vi "Dropout Voltage.vi"() -> ()   [LabVIEW 2020]
doc: "Demonstrates how to use triggers and events to synchronize multiple channels in Sequence source mode. Use this example to sequence multiple channels in lock-step."
uses:
  <instrlib>/niDCPower/nidcpower.llb/niDCPower Output Function.ctl
  <instrlib>/niDCPower/nidcpower.llb/niDCPower Source Mode.ctl
  <instrlib>/niDCPower/nidcpower.llb/niDCPower Sequence Attribute Type.ctl
  <instrlib>/niDCPower/nidcpower.llb/niDCPower Wait For Event - Event.ctl
  <instrlib>/niDCPower/nidcpower.llb/niDCPower Sense.ctl
  <instrlib>/niDCPower/nidcpower.llb/niDCPower Create Advanced Sequence Step.vi
  <instrlib>/niDCPower/nidcpower.llb/niDCPower Disable Source Trigger.vi
  <instrlib>/niDCPower/nidcpower.llb/niDCPower Configure Digital Edge Source Trigger.vi
  <instrlib>/niDCPower/nidcpower.llb/niDCPower Configure Digital Edge Measure Trigger.vi
panel:
  in  "Aperture time (s)":dbl=0.1
  in  "DUT setup time (s)":dbl
  out "Input Voltage (V) vs. Output Voltage (V)":T1(graph) caption="Current (Amps) vs Voltage (Volts)"
  in  "Load device wait (s)":dbl=0.1
  in  "Sweep type":u16(ring) items=["Linear", "Logarithmic"]
  in  "Load device max. voltage (V)":dbl=20.0
  in  "Load values (A)":dbl[](array[numeric])=[0.01, 0.1, 1.0, 2.5] min=0.0
  in  "Timeout (s)":dbl=30.0 format="%.3p"
  in  "Source device name":refnum<k15>="PXI2Slot2"
  in  "Load device source delay (s)":dbl=0.1
  in  "Source device current limit (A)":dbl=25.0
  in  "Load device max. sink power (W)":dbl=300.0
  in  "Source device channel":string="0"
  in  "Load device channel":string="0"
  in  "Points or Points/Decade":i32=21 min=1
  in  "Voltage source level stop":dbl=3.0 caption="Current load level stop" min=0.0 step=0.1
  in  "Voltage source level start":dbl=6.5 min=0.0 step=0.1
  in  "Load device name":refnum<k15>="PXI2Slot4"
  # "Source config"
  # "Load Config"
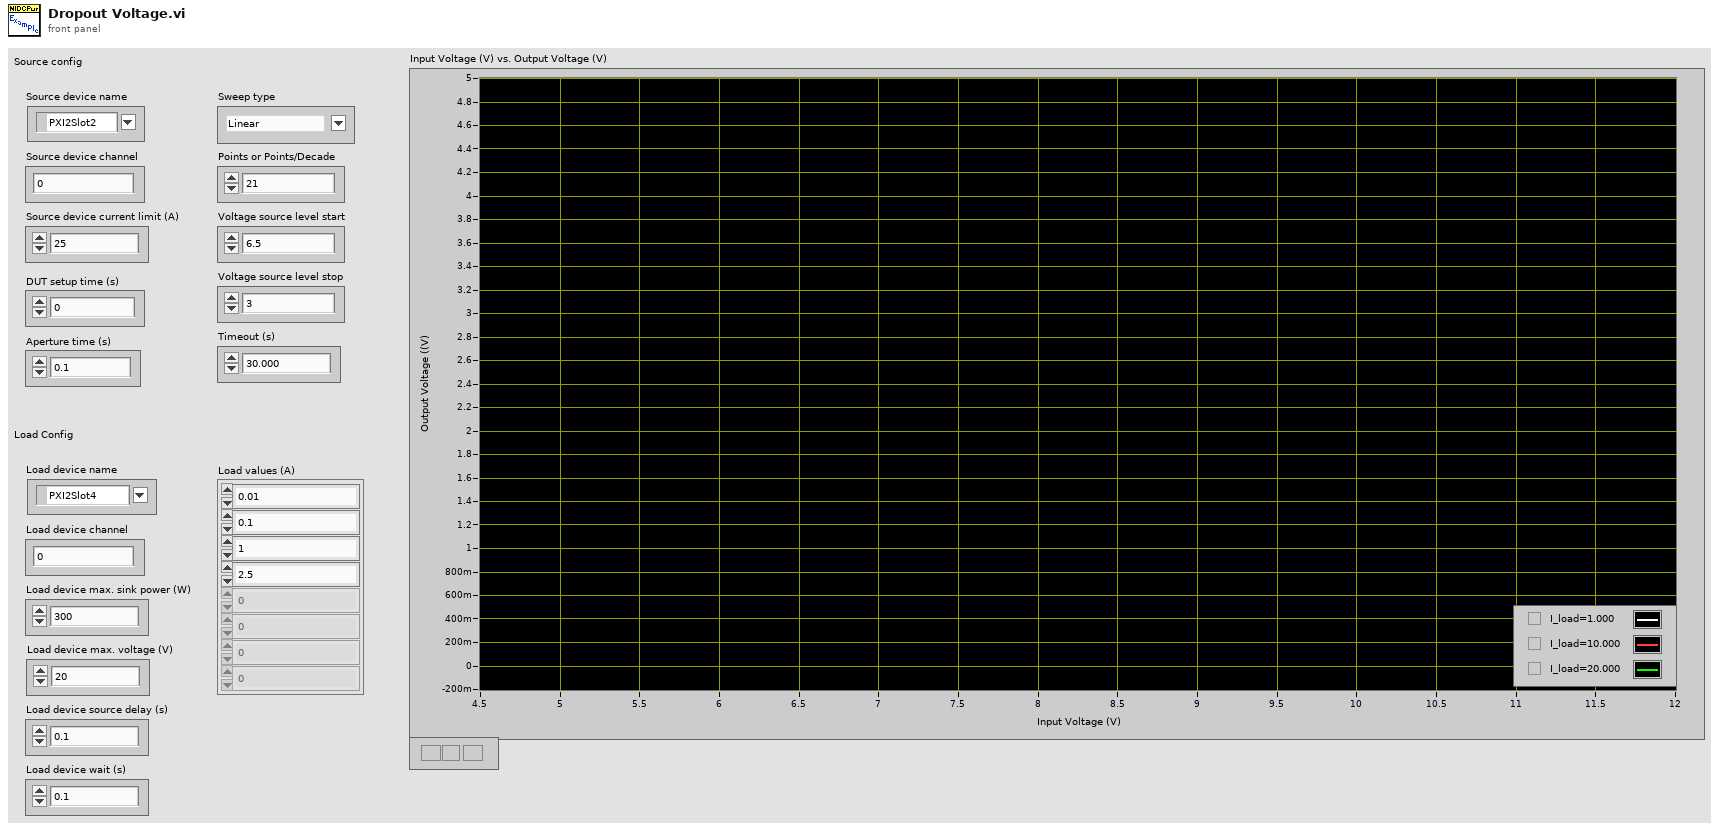
[diagram p1: front panel]
types:
  T1 = cluster{"voltage measurements":dbl[], "current measurements":dbl[]}[]
  T2 = typedef "niDCPower Wait For Event - Event.ctl" = i32
  T3 = typedef "niDCPower Source Mode.ctl" = i32
  T4 = typedef "niDCPower Sense.ctl" = i32
  T5 = typedef "niDCPower Sequence Attribute Type.ctl" = i32
  T6 = typedef "niDCPower Output Function.ctl" = i32
  T7 = cluster{"voltage measurements":dbl[], "voltage measurements":dbl[]}
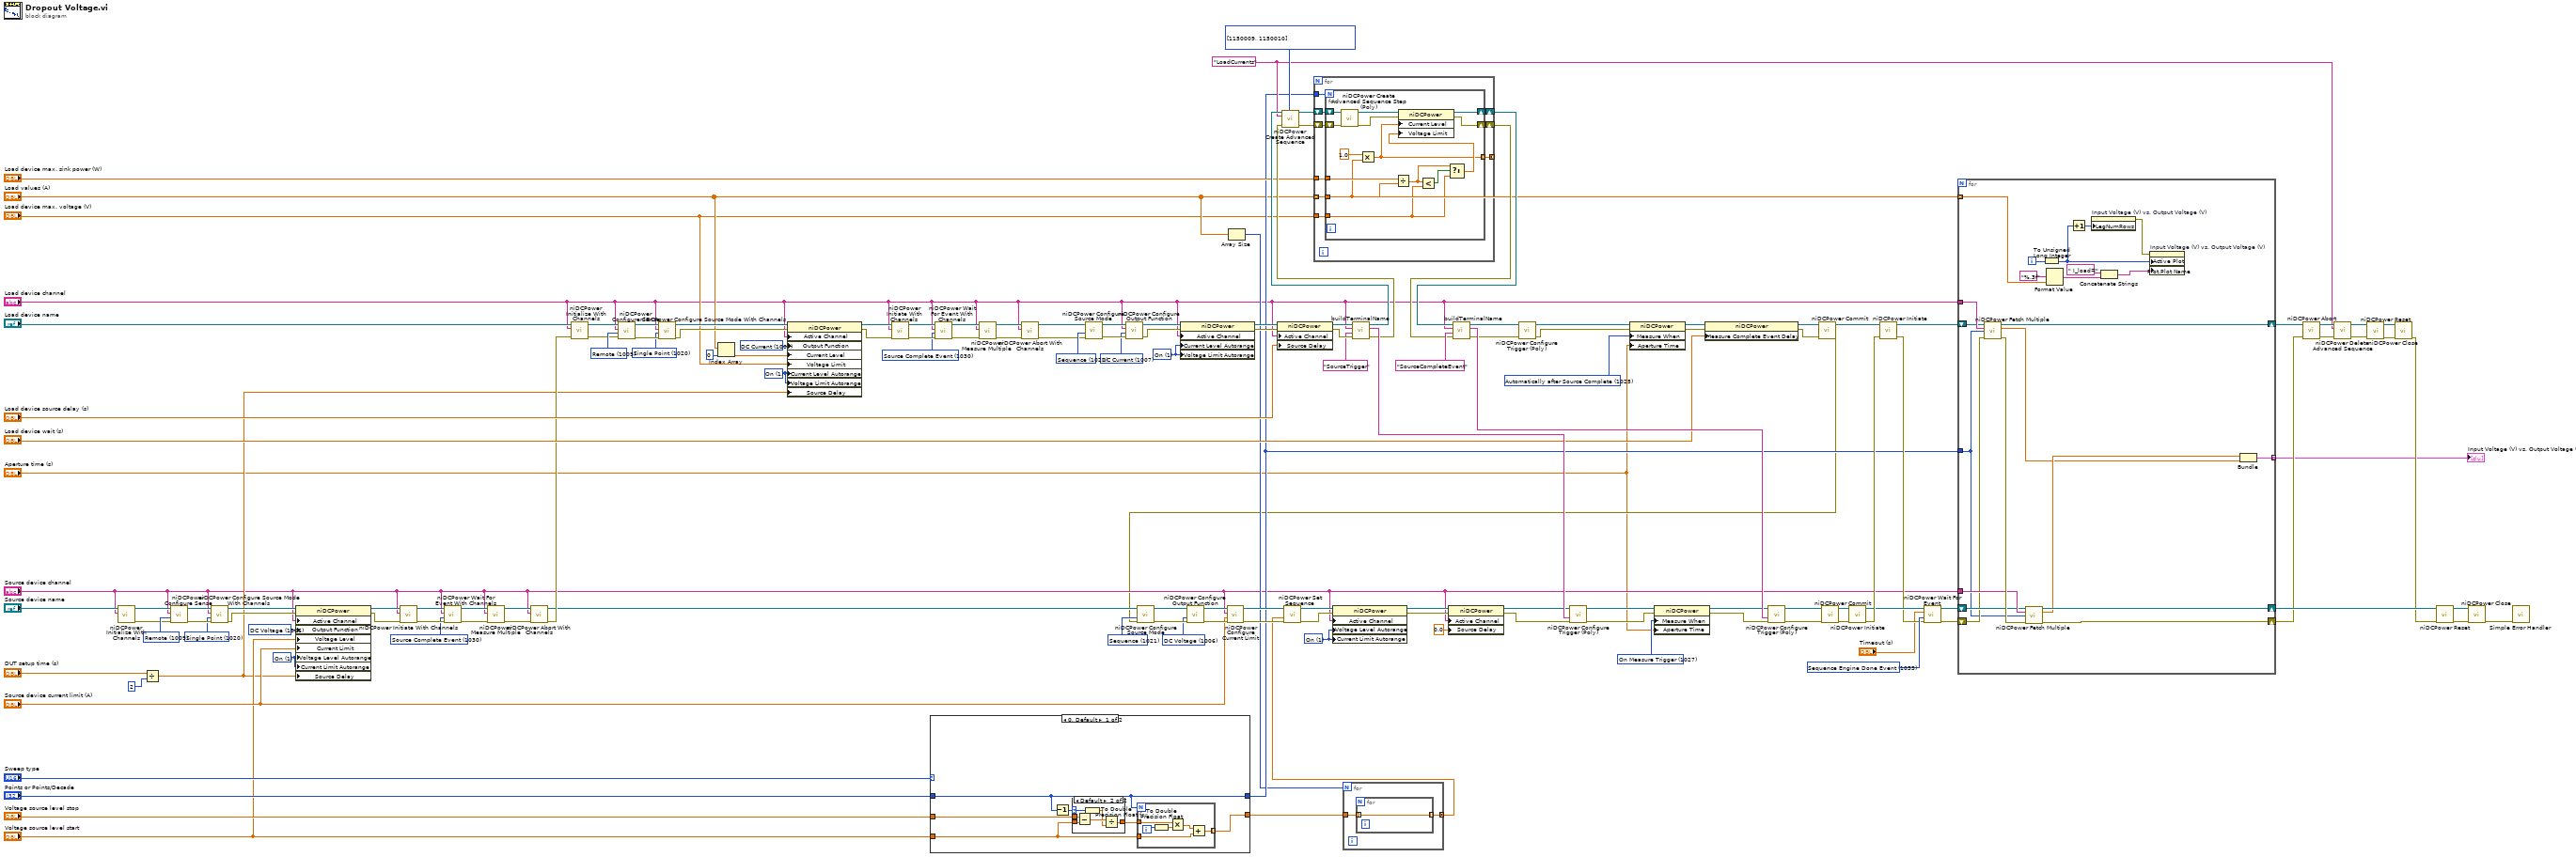
[diagram p0: block diagram]
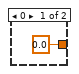
[diagram p2: hidden frame]
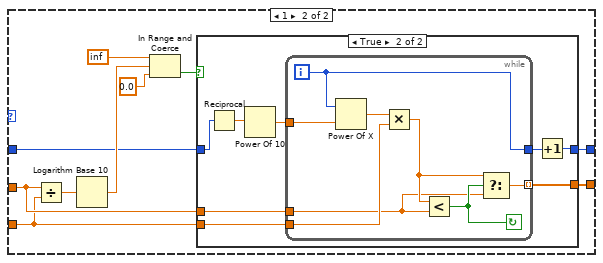
[diagram p3: hidden frame]
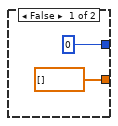
[diagram p4: hidden frame]
diagram:
  w1 = 1025 items=["Automatically after Source Complete"=1025, "On Demand"=1026, "On Measure Trigger"=1027] ("Measurement:Advanced:Measure When")
  w20 = T2 1030 items=["Source Complete Event"=1030, "Measure Complete Event"=1031, "Sequence Iteration Complete Event"=1032, "Sequence Engine Done Event"=1033, "Pulse Complete Event"=1051, "Ready For Pulse Trigger Event"=1052] ("event")
  w25 = 1 items=["Off", "On"] ("Source:DC Current:Current Level Autorange")
  w26 = 1007 items=["DC Voltage"=1006, "DC Current"=1007, "Pulse Voltage"=1049, "Pulse Current"=1050] ("Source:Output Function")
  w27 = T3 1020 items=["Single Point"=1020, "Sequence"=1021] ("source mode")
  w32 = T4 1009 items=["Local"=1008, "Remote"=1009] ("sense")
  w44 = T2 1030 items=["Source Complete Event"=1030, "Measure Complete Event"=1031, "Sequence Iteration Complete Event"=1032, "Sequence Engine Done Event"=1033, "Pulse Complete Event"=1051, "Ready For Pulse Trigger Event"=1052] ("event")
  w49 = 1 items=["Off", "On"] ("Source:DC Current:Current Level Autorange")
  w50 = 1006 items=["DC Voltage"=1006, "DC Current"=1007, "Pulse Voltage"=1049, "Pulse Current"=1050] ("Source:Output Function")
  w51 = T3 1020 items=["Single Point"=1020, "Sequence"=1021] ("source mode")
  w56 = T4 1009 items=["Local"=1008, "Remote"=1009] ("sense")
  w91 = T2 1033 items=["Source Complete Event"=1030, "Measure Complete Event"=1031, "Sequence Iteration Complete Event"=1032, "Sequence Engine Done Event"=1033] ("event")
  w96 = 1 items=["Off", "On"] ("DC Voltage:Voltage Level Autorange")
  w110 = 1 items=["Off", "On"] ("DC Voltage:Voltage Level Autorange")
  w111 = T5[] [1150009, 1150010] items=["Source -> Output Function"=1150008, "Source -> Output Enabled"=1250006, "Source -> Output Resistance"=1150061, "Source -> Transient Response"=1150062, "Source -> Custom Transient Response -> Voltage Gain Bandwidth"=1150067, "Source -> Custom Transient Response -> Voltage Compensation Frequency"=1150068, "Source -> Custom Transient Response -> Voltage Pole-Zero Ratio"=1150069, "Source -> Custom Transient Response -> Current Gain Bandwidth"=1150070, "Source -> Custom Transient Response -> Current Compensation Frequency"=1150071, "Source -> Custom Transient Response -> Current Pole-Zero Ratio"=1150072, "Source -> DC Voltage -> Voltage Level"=1250001, "Source -> DC Voltage -> Voltage Level Range"=1150005, "Source -> DC Voltage -> Current Limit"=1250005, "Source -> DC Voltage -> Current Limit High"=1150187, "Source -> DC Voltage -> Current Limit Low"=1150188, "Source -> DC Voltage -> Current Limit Range"=1150004, "Source -> DC Current -> Current Level"=1150009, "Source -> DC Current -> Current Level Range"=1150011, "Source -> DC Current -> Voltage Limit"=1150010, "Source -> DC Current -> Voltage Limit High"=1150185, "Source -> DC Current -> Voltage Limit Low"=1150186, "Source -> DC Current -> Voltage Limit Range"=1150012, "Source -> Pulse Voltage -> Pulse Voltage Level"=1150080, "Source -> Pulse Voltage -> Pulse Bias Voltage Level"=1150082, "Source -> Pulse Voltage -> Pulse Voltage Level Range"=1150084, "Source -> Pulse Voltage -> Pulse Current Limit"=1150081, "Source -> Pulse Voltage -> Pulse Current Limit High"=1150193, "Source -> Pulse Voltage -> Pulse Current Limit Low"=1150194, "Source -> Pulse Voltage -> Pulse Bias Current Limit"=1150083, "Source -> Pulse Voltage -> Pulse Bias Current Limit High"=1150195, "Source -> Pulse Voltage -> Pulse Bias Current Limit Low"=1150196, "Source -> Pulse Voltage -> Pulse Current Limit Range"=1150085, "Source -> Pulse Current -> Pulse Current Level"=1150086, "Source -> Pulse Current -> Pulse Bias Current Level"=1150088, "Source -> Pulse Current -> Pulse Current Level Range"=1150090, "Source -> Pulse Current -> Pulse Voltage Limit"=1150087, "Source -> Pulse Current -> Pulse Voltage Limit High"=1150189, "Source -> Pulse Current -> Pulse Voltage Limit Low"=1150190, "Source -> Pulse Current -> Pulse Bias Voltage Limit"=1150089, "Source -> Pulse Current -> Pulse Bias Voltage Limit High"=1150191, "Source -> Pulse Current -> Pulse Bias Voltage Limit Low"=1150192, "Source -> Pulse Current -> Pulse Voltage Limit Range"=1150091, "Source -> Advanced -> Source Delay"=1150051, "Source -> Advanced -> Pulse Bias Delay"=1150092, "Source -> Advanced -> Pulse On Time"=1150093, "Source -> Advanced -> Pulse Off Time"=1150094, "Source -> Advanced -> OVP Enabled"=1250002, "Source -> Advanced -> OVP Limit"=1250003, "Source -> Advanced -> Compliance Limit Symmetry"=1150184, "Source -> Advanced -> Sequence Step Delta Time"=1150198, "Measurement -> Sense"=1150013, "Measurement -> Aperture Time"=1150058, "Measurement -> Measure Record Length"=1150063, "Measurement -> Advanced -> DC Noise Rejection"=1150066, "Measurement -> Autorange"=1150244, "Measurement -> Advanced -> Autorange Behavior"=1150245, "Measurement -> Advanced -> Autorange Aperture Time Mode"=1150246, "Measurement -> Advanced -> Autorange Minimum Aperture Time"=1150247, "Measurement -> Advanced -> Autorange Minimum Aperture Time Units"=1150248, "Measurement -> Advanced -> Autorange Minimum Current Range"=1150255, "Measurement -> Advanced -> Autorange Minimum Voltage Range"=1150256, "Measurement -> Advanced -> Autorange Threshold Mode"=1150257, "Measurement -> Advanced -> Autorange Maximum Delay After Range Change"=1150322, "LCR -> Instrument Mode"=1150208, "LCR -> LCR Stimulus Function"=1150209, "LCR -> LCR Frequency"=1150210, "LCR -> LCR Voltage Amplitude"=1150211, "LCR -> LCR Current Amplitude"=1150212, "LCR -> LCR DC Bias Source"=1150213, "LCR -> LCR DC Bias Voltage Level"=1150214, "LCR -> LCR DC Bias Current Level"=1150215, "LCR -> LCR Impedance Autorange"=1150216, "LCR -> LCR Impedance Range"=1150217, "LCR -> LCR Measurement Time"=1150218, "LCR -> LCR Custom Measurement Time"=1150258, "LCR -> LCR Source Delay Mode"=1150315, "LCR -> Compensation -> Open -> Enabled"=1150220, "LCR -> Compensation -> Open -> Conductance"=1150261, "LCR -> Compensation -> Open -> Susceptance"=1150262, "LCR -> Compensation -> Short -> Enabled"=1150221, "LCR -> Compensation -> Short -> Resistance"=1150263, "LCR -> Compensation -> Short -> Reactance"=1150264, "LCR -> Compensation -> Load -> Enabled"=1150222, "LCR -> Compensation -> Load -> Measured Resistance"=1150268, "LCR -> Compensation -> Load -> Measured Reactance"=1150269, "LCR -> Compensation -> Load -> Actual Resistance"=1150270, "LCR -> Compensation -> Load -> Actual Reactance"=1150271] ("advanced sequence properties")
  w76 = "LoadCurrents" ("sequence name")
  w116 = T6 1006 items=["DC Voltage"=1006, "DC Current"=1007, "Pulse Voltage"=1049, "Pulse Current"=1050] ("output function")
  w117 = 1027 items=["Automatically after Source Complete"=1025, "On Demand"=1026, "On Measure Trigger"=1027] ("Measurement:Advanced:Measure When")
  w118 = T3 1021 items=["Single Point"=1020, "Sequence"=1021] ("source mode")
  w125 = T6 1007 items=["DC Voltage"=1006, "DC Current"=1007, "Pulse Voltage"=1049, "Pulse Current"=1050] ("output function")
  w139 = T3 1021 items=["Single Point"=1020, "Sequence"=1021] ("source mode")
  n1 = call <instrlib>:"niDCPower Initialize With Channels.vi"("channels"="Source device channel", "resource name"="Source device name") -> ("error out"=w37:errorcluster, "instrument handle out"=w38:refnum<k15>)  [unwired: 3 in, 5 out]
  n2 = Divide(x="DUT setup time (s)", y=2) -> (x/y=w12:dbl)
  n3 = call <instrlib>:"niDCPower Configure Sense.vi"("error in (no error)"=w37, "sense"=w56, "channel name"="Source device channel", "instrument handle"=w38) -> ("error out"=w52:errorcluster, "instrument handle out"=w53:refnum<k15>)  [unwired: 6 in]
  n4 = call <instrlib>:"niDCPower Configure Source Mode With Channels.vi"("error in (no error)"=w52, "source mode"=w51, "channel name"="Source device channel", "instrument handle"=w53) -> ("error out"=w55:errorcluster, "instrument handle out"=w54:refnum<k15>)  [unwired: 6 in]
  n5 = property class="niDCPower"(reference=w54, error in=w55, "Active Channel"="Source device channel", "Output Function"=w50, "Voltage Level"="Voltage source level start", "Current Limit"="Source device current limit (A)", "Voltage Level Autorange"=w49, "Current Limit Autorange"=w49, "Source Delay"=w12) -> (reference out=w48:refnum<k15>, error out=w47:errorcluster)
  n6 = call <instrlib>:"niDCPower Initiate With Channels.vi"("error in (no error)"=w47, "channel name"="Source device channel", "instrument handle"=w48) -> ("error out"=w45:errorcluster, "instrument handle out"=w46:refnum<k15>)  [unwired: 7 in]
  n7 = call <instrlib>:"niDCPower Wait For Event With Channels.vi"("error in (no error)"=w45, "event"=w44, "channel name"="Source device channel", "instrument handle"=w46) -> ("error out"=w43:errorcluster, "instrument handle out"=w42:refnum<k15>)  [unwired: 6 in]
  n8 = call <instrlib>:"niDCPower Measure Multiple.vi"("error in (no error)"=w43, "channel name"="Source device channel", "instrument handle"=w42) -> ("error out"=w40:errorcluster, "instrument handle out"=w39:refnum<k15>)  [unwired: 5 in, 2 out]
  n9 = call <instrlib>:"niDCPower Abort With Channels.vi"("error in (no error)"=w40, "channel name"="Source device channel", "instrument handle"=w39) -> ("error out"=w33:errorcluster, "instrument handle out"=w6:refnum<k15>)  [unwired: 7 in]
  n10 = call <instrlib>:"niDCPower Initialize With Channels.vi"("error in (no error)"=w33, "channels"="Load device channel", "resource name"="Load device name") -> ("error out"=w13:errorcluster, "instrument handle out"=w14:refnum<k15>)  [unwired: 2 in, 5 out]
  n11 = call <instrlib>:"niDCPower Configure Sense.vi"("error in (no error)"=w13, "sense"=w32, "channel name"="Load device channel", "instrument handle"=w14) -> ("error out"=w28:errorcluster, "instrument handle out"=w29:refnum<k15>)  [unwired: 6 in]
  n12 = call <instrlib>:"niDCPower Configure Source Mode With Channels.vi"("error in (no error)"=w28, "source mode"=w27, "channel name"="Load device channel", "instrument handle"=w29) -> ("error out"=w31:errorcluster, "instrument handle out"=w30:refnum<k15>)  [unwired: 6 in]
  n13 = Index Array(array="Load values (A)", index=0) -> (element=w10:dbl)
  n14 = property class="niDCPower"(reference=w30, error in=w31, "Active Channel"="Load device channel", "Output Function"=w26, "Current Level"=w10, "Voltage Limit"="Load device max. voltage (V)", "Current Level Autorange"=w25, "Voltage Limit Autorange"=w25, "Source Delay"=w12) -> (reference out=w24:refnum<k15>, error out=w23:errorcluster)
  n15 = call <instrlib>:"niDCPower Initiate With Channels.vi"("error in (no error)"=w23, "channel name"="Load device channel", "instrument handle"=w24) -> ("error out"=w21:errorcluster, "instrument handle out"=w22:refnum<k15>)  [unwired: 7 in]
  n16 = case shown="0, Default" "Sweep type" {
    tunnel: "Points or Points/Decade" -> [w148 w167]
    tunnel: [w151 w171] -> w61
    tunnel: "Voltage source level start" -> [w150 w168]
    tunnel: "Voltage source level stop" -> [w149 w175]
    tunnel: [w148 w172] -> w73
    frame 0, Default {
      n17 = Decrement(x=w148) -> (x-1=w153:i32)
      n18 = case shown="Default" w153 {
        selector: w153 -> [_ w161]
        tunnel: w149 -> [_ w166]
        tunnel: w150 -> [_ w165]
        tunnel: [0.0 w163] -> w152
        frame 0 {
        }
        frame Default {
          n19 = Subtract(x=w166, y=w165) -> (x-y=w164:dbl)
          n20 = To Double Precision Float(number=w161) -> (double precision float=w162:dbl)
          n21 = Divide(x=w164, y=w162) -> (x/y=w163:dbl)
        }
      }
      n22 = for {
        N: w148 -> [_]
        tunnel: w152 -> [w158]
        tunnel: w150 -> [w159]
        tunnel: [w154] -> w151 mode=indexing
        i -> [w157]
        n23 = To Double Precision Float(number=w157) -> (double precision float=w155:dbl)
        n24 = Multiply(x=w158, y=w155) -> (x*y=w156:dbl)
        n25 = Add(x=w156, y=w159) -> (x+y=w154:dbl)
      }
    }
    frame 1 {
      n26 = Divide(x=w175, y=w168) -> (x/y=w176:dbl)
      n27 = Logarithm Base 10(1:w176) -> (0:w173:dbl)
      n28 = In Range and Coerce(upper limit=inf, x=w173, lower limit=0.0) -> (In Range?=w170:bool)  [unwired: 1 out]
      n29 = case shown="True" w170 {
        tunnel: [dbl[] [] w186] -> w171
        tunnel: [0 w179] -> w172
        tunnel: w175 -> [_ w185]
        tunnel: w168 -> [_ w184]
        tunnel: w167 -> [_ w181]
        frame False {
        }
        frame True {
          n30 = Reciprocal(x=w181) -> (1/x=w183:dbl)
          n31 = Power Of 10(x=w183) -> (10^x=w182:dbl)
          n32 = while {
            tunnel: w182 -> [w191]
            tunnel: w184 -> [w194]
            tunnel: [w190] -> w186 mode=indexing
            tunnel: [w192] -> w180
            tunnel: w185 -> [w187]
            i -> [w192]
            stop <- w189 continue-if-true
            n33 = Power Of X(1:w191, 2:w192) -> (0:w193:dbl)
            n34 = Multiply(x=w193, y=w194) -> (x*y=w188:dbl)
            n35 = Less?(x=w188, y=w187) -> (x < y?=w189:bool)
            n36 = Select(t=w188, s=w189, f=w187) -> (s? t:f=w190:dbl)
          }
          n37 = Increment(x=w180) -> (x+1=w179:i32)
        }
      }
    }
  }
  n38 = call <instrlib>:"niDCPower Wait For Event With Channels.vi"("error in (no error)"=w21, "event"=w20, "channel name"="Load device channel", "instrument handle"=w22) -> ("error out"=w19:errorcluster, "instrument handle out"=w18:refnum<k15>)  [unwired: 6 in]
  n39 = call <instrlib>:"niDCPower Measure Multiple.vi"("error in (no error)"=w19, "channel name"="Load device channel", "instrument handle"=w18) -> ("error out"=w17:errorcluster, "instrument handle out"=w16:refnum<k15>)  [unwired: 5 in, 2 out]
  n40 = call <instrlib>:"niDCPower Abort With Channels.vi"("error in (no error)"=w17, "channel name"="Load device channel", "instrument handle"=w16) -> ("error out"=w7:errorcluster, "instrument handle out"=w8:refnum<k15>)  [unwired: 7 in]
  n41 = call <instrlib>:"niDCPower Configure Source Mode.vi"("error in (no error)"=w7, "source mode"=w139, "instrument handle"=w8) -> ("error out"=w141:errorcluster, "instrument handle out"=w140:refnum<k15>)  [unwired: 7 out]
  n42 = call <instrlib>:"niDCPower Configure Output Function.vi"("error in (no error)"=w141, "output function"=w125, "channel name"="Load device channel", "instrument handle"=w140) -> ("error out"=w57:errorcluster, "instrument handle out"=w58:refnum<k15>)  [unwired: 6 out]
  n43 = property class="niDCPower"(reference=w58, error in=w57, "Active Channel"="Load device channel", "Current Level Autorange"=w110, "Voltage Limit Autorange"=w110) -> (reference out=w108:refnum<k15>, error out=w107:errorcluster)
  n44 = Array Size(array="Load values (A)") -> (size(s)=w66:i32)
  n45 = property class="niDCPower"(reference=w108, error in=w107, "Active Channel"="Load device channel", "Source Delay"="Load device source delay (s)") -> (reference out=w133:refnum<k15>, error out=w131:errorcluster)
  n46 = for {
    N: w66 -> [_]
    tunnel: w61 -> [w196]
    tunnel: [w195] -> w67 mode=concatenating
    n47 = for {
      tunnel: w196 -> [w197] mode=indexing
      tunnel: [w197] -> w195 mode=indexing
    }
  }
  n48 = call "buildTerminalName.vi"("error in (no error)"=w131, "Local Terminal Name"="SourceTrigger", "Channel Name"="Load device channel", "session handle"=w133) -> ("error IO"=w103:errorcluster, "Fully Qualified Terminal Name"=w129:string, "session handle 2"=w105:refnum<k15>)  [unwired: 5 out]
  n49 = call <instrlib>:"niDCPower Create Advanced Sequence.vi"("instrument handle"=w105, "sequence name"=w76, "advanced sequence properties"=w111, "error in (no error)"=w103) -> ("instrument handle out"=w113:refnum<k15>, "error out"=w112:errorcluster)  [unwired: 10 in]
  n50 = for {
    tunnel: "Load device max. sink power (W)" -> [w202]
    tunnel: "Load device max. voltage (V)" -> [w201]
    tunnel: "Load values (A)" -> [w200] mode=indexing
    shift-right: [w204] -> w104
    shift-left: w113 -> [w206]
    shift-right: [w203] -> w102
    shift-left: w112 -> [w205]
    tunnel: w73 -> [w199]
    tunnel: [w198] -> _ mode=concatenating
    n51 = for {
      N: w199 -> [_]
      shift-right: [w217] -> w203
      shift-left: w205 -> [w220]
      shift-right: [w216] -> w204
      shift-left: w206 -> [w215]
      tunnel: w202 -> [w214]
      tunnel: w200 -> [w209]
      tunnel: w201 -> [w212]
      tunnel: [w207] -> w198 mode=indexing
      n52 = call-poly <instrlib>:"niDCPower Create Advanced Sequence Step (Poly).vi"("error in (no error)"=w220, "instrument handle"=w215) -> ("error out"=w218:errorcluster, "instrument handle out"=w219:refnum<k15>)  [unwired: 8 in]
      n53 = Multiply(x=1.0, y=w209) -> (x*y=w207:dbl)
      n54 = Divide(x=w214, y=w209) -> (x/y=w211:dbl)
      n55 = Less?(x=w211, y=w212) -> (x < y?=w213:bool)
      n56 = Select(t=w211, s=w213, f=w212) -> (s? t:f=w210:dbl)
      n57 = property class="niDCPower"(reference=w219, error in=w218, "Current Level"=w207, "Voltage Limit"=w210) -> (reference out=w216:refnum<k15>, error out=w217:errorcluster)
    }
  }
  n58 = call "buildTerminalName.vi"("error in (no error)"=w102, "Local Terminal Name"="SourceCompleteEvent", "Channel Name"="Load device channel", "session handle"=w104) -> ("error IO"=w127:errorcluster, "Fully Qualified Terminal Name"=w128:string, "session handle 2"=w132:refnum<k15>)  [unwired: 5 out]
  n59 = call-poly <instrlib>:"niDCPower Configure Trigger (Poly).vi"("error in (no error)"=w127, "instrument handle"=w132) -> ("error out"=w142:errorcluster, "instrument handle out"=w143:refnum<k15>)  [unwired: 1 in, 7 out]
  n60 = property class="niDCPower"(reference=w143, error in=w142, "Measure When"=w1, "Aperture Time"="Aperture time (s)") -> (reference out=w137:refnum<k15>, error out=w134:errorcluster)
  n61 = property class="niDCPower"(reference=w137, error in=w134, "Measure Complete Event Delay"="Load device wait (s)") -> (reference out=w136:refnum<k15>, error out=w135:errorcluster)
  n62 = call <instrlib>:"niDCPower Commit.vi"("error in (no error)"=w135, "instrument handle"=w136) -> ("error out"=w3:errorcluster, "instrument handle out"=w63:refnum<k15>)  [unwired: 8 out]
  n63 = call <instrlib>:"niDCPower Configure Source Mode.vi"("error in (no error)"=w3, "source mode"=w118, "instrument handle"=w6) -> ("error out"=w120:errorcluster, "instrument handle out"=w119:refnum<k15>)  [unwired: 7 out]
  n64 = call <instrlib>:"niDCPower Configure Output Function.vi"("error in (no error)"=w120, "output function"=w116, "instrument handle"=w119) -> ("error out"=w60:errorcluster, "instrument handle out"=w59:refnum<k15>)  [unwired: 1 in, 6 out]
  n65 = call <instrlib>:"niDCPower Configure Current Limit.vi"("error in (no error)"=w60, "current limit"="Source device current limit (A)", "channel name"="Source device channel", "instrument handle"=w59) -> ("error out"=w92:errorcluster, "instrument handle out"=w93:refnum<k15>)  [unwired: 6 in]
  n66 = call <instrlib>:"niDCPower Set Sequence.vi"("error in (no error)"=w92, "values"=w67, "instrument handle"=w93) -> ("error out"=w68:errorcluster, "instrument handle out"=w69:refnum<k15>)  [unwired: 2 in, 5 out]
  n67 = property class="niDCPower"(reference=w69, error in=w68, "Active Channel"="Source device channel", "Voltage Level Autorange"=w96, "Current Limit Autorange"=w96) -> (reference out=w95:refnum<k15>, error out=w94:errorcluster)
  n68 = property class="niDCPower"(reference=w95, error in=w94, "Active Channel"="Source device channel", "Source Delay"=0.0 ("Source:Advanced:Source Delay")) -> (reference out=w71:refnum<k15>, error out=w70:errorcluster)
  n69 = call-poly <instrlib>:"niDCPower Configure Trigger (Poly).vi"("error in (no error)"=w70, "input terminal"=w129, "instrument handle"=w71) -> ("error out"=w123:errorcluster, "instrument handle out"=w124:refnum<k15>)  [unwired: 1 in, 6 out]
  n70 = property class="niDCPower"(reference=w124, error in=w123, "Measure When"=w117, "Aperture Time"="Aperture time (s)") -> (reference out=w121:refnum<k15>, error out=w122:errorcluster)
  n71 = call-poly <instrlib>:"niDCPower Configure Trigger (Poly).vi"("error in (no error)"=w122, "input terminal"=w128, "instrument handle"=w121) -> ("error out"=w65:errorcluster, "instrument handle out"=w64:refnum<k15>)  [unwired: 1 in, 6 out]
  n72 = call <instrlib>:"niDCPower Commit.vi"("error in (no error)"=w65, "instrument handle"=w64) -> ("error out"=w145:errorcluster, "instrument handle out"=w146:refnum<k15>)  [unwired: 8 out]
  n73 = call <instrlib>:"niDCPower Initiate.vi"("error in (no error)"=w145, "instrument handle"=w146) -> ("error out"=w138:errorcluster, "instrument handle out"=w90:refnum<k15>)  [unwired: 8 out]
  n74 = call <instrlib>:"niDCPower Initiate.vi"("error in (no error)"=w138, "instrument handle"=w63) -> ("error out"=w88:errorcluster, "instrument handle out"=w86:refnum<k15>)  [unwired: 8 out]
  n75 = call <instrlib>:"niDCPower Wait For Event.vi"("timeout (10.0)"="Timeout (s)", "error in (no error)"=w88, "event"=w91, "instrument handle"=w90) -> ("error out"=w87:errorcluster, "instrument handle out"=w89:refnum<k15>)  [unwired: 6 out]
  n76 = for {
    tunnel: "Source device channel" -> [w240]
    tunnel: "Load device channel" -> [w239]
    shift-right: [w242] -> w144
    shift-left: w89 -> [w238]
    shift-right: [w234] -> w78
    shift-left: w87 -> [w237]
    shift-right: [w235] -> w79
    shift-left: w86 -> [w236]
    tunnel: w73 -> [w223]
    tunnel: "Load values (A)" -> [w230] mode=indexing
    tunnel: [w224] -> w75 mode=indexing
    i -> [w225]
    n77 = call <instrlib>:"niDCPower Fetch Multiple.vi"("instrument handle"=w236, "channel name"=w239, "count (1)"=w223, "error in (no error)"=w237) -> ("instrument handle out"=w235:refnum<k15>, "voltage measurements"=w221:dbl[], "error out"=w241:errorcluster)  [unwired: 1 in, 8 out]
    n78 = call <instrlib>:"niDCPower Fetch Multiple.vi"("instrument handle"=w238, "channel name"=w240, "count (1)"=w223, "error in (no error)"=w241) -> ("instrument handle out"=w242:refnum<k15>, "voltage measurements"=w222:dbl[], "error out"=w234:errorcluster)  [unwired: 1 in, 8 out]
    n79 = To Unsigned Long Integer(number=w225) -> (unsigned 32bit integer=w229:u32)
    n80 = Format Value(format string="%.3f", value (0)=w230) -> (output string=w231:string)  [unwired: 1 out]
    n81 = Increment(x=w229) -> (x+1=w227:u32)
    n82 = property on="Input Voltage (V) vs. Output Voltage (V)" class="XYGraph (strict)"("LegNumRows"=w227) -> (error out=w226:errorcluster)  [unwired: 2 in, 1 out]
    n83 = Concatenate Strings(" I_load=" ("string"), w231) -> (w228:string)
    n84 = property on="Input Voltage (V) vs. Output Voltage (V)" class="XYGraph (strict)"(error in=w226, "Active Plot"=w229, "Plot.Plot Name"=w228) -> ()  [unwired: 1 in, 2 out]
    n85 = Bundle("voltage measurements"=w222, "voltage measurements"=w221) -> (w224:T7)  [unwired: 1 out]
  }
  "Input Voltage (V) vs. Output Voltage (V)" <- w75
  n86 = call <instrlib>:"niDCPower Abort.vi"("error in (no error)"=w78, "instrument handle"=w79) -> ("error out"=w81:errorcluster, "instrument handle out"=w82:refnum<k15>)  [unwired: 8 in]
  n87 = call <instrlib>:"niDCPower Delete Advanced Sequence.vi"("error in (no error)"=w81, "sequence name"=w76, "instrument handle"=w82) -> ("error out"=w80:errorcluster, "instrument handle out"=w83:refnum<k15>)  [unwired: 7 in]
  n88 = call <instrlib>:"niDCPower Reset.vi"("error in (no error)"=w80, "instrument handle"=w83) -> ("error out"=w84:errorcluster, "instrument handle out"=w85:refnum<k15>)  [unwired: 2 in, 6 out]
  n89 = call <instrlib>:"niDCPower Close.vi"("error in (no error)"=w84, "instrument handle"=w85) -> ("error out"=w77:errorcluster)  [unwired: 9 out]
  n90 = call <instrlib>:"niDCPower Reset.vi"("error in (no error)"=w77, "instrument handle"=w144) -> ("error out"=w115:errorcluster, "instrument handle out"=w114:refnum<k15>)  [unwired: 1 in, 7 out]
  n91 = call <instrlib>:"niDCPower Close.vi"("error in (no error)"=w115, "instrument handle"=w114) -> ("error out"=w147:errorcluster)  [unwired: 9 out]
  n92 = call <vilib>:"Simple Error Handler.vi"("error in (no error)"=w147) -> ()  [unwired: 1 in, 8 out]
